vi "Dialog Data Entry.vi"   [LabVIEW 2012]
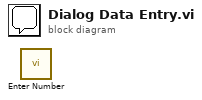
[diagram p0: block diagram]
diagram:
  n1 = call "Enter Number.vi"() -> ()  [unwired: 10 in, 2 out]
